vi "libssh2_channel_flush_ex.vi"(8 "error in (no error)":errorcluster, 10 "streamid":i32, 11 "channel":u64) -> (0 "error out":errorcluster, 3 "return value":i32)   [LabVIEW 2013, in "libssh2.lvlib"]
uses:
  libssh2.lvlib
  libssh2.dll
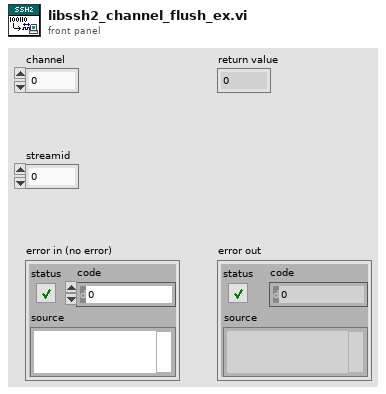
[diagram p1: front panel]
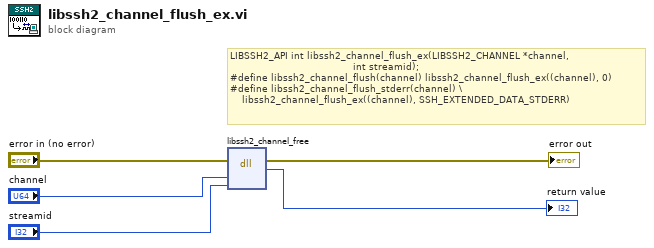
[diagram p0: block diagram]
diagram:
  # "LIBSSH2_API int libssh2_channel_flush_ex(LIBSSH2_CHANNEL *channel,\n                                         int streamid);\n#define libssh2_channel_flush(channel) libssh2_channel_flush_ex((channel), 0)\n#define libssh2_channel_flush_stderr(channel) \\\n    libssh2_channel_flush_ex((channel), SSH_EXTENDED_DATA_STDERR)"
  n1 = dll-call lib="C:/Users/pasca/source/repos/libssh2-labview/libssh2**.*" fn="libssh2_channel_free"(error in="error in (no error)", "channel"="channel", "streamid"="streamid") -> (error out=→"error out":errorcluster, "return value"=→"return value":i32)  [unwired: 4 in, 1 out]
